vi "Get All Sub-Entries.vi"(8 "Error In":errorcluster, 11 "reference in":refnum<class "OD Entry.lvclass">) -> (0 "Error Out":errorcluster, 1 "Indices":u8[](array[numeric]), 2 "Sub-Entries":refnum<class "OD Sub-Entry.lvclass">[](array[class]), 3 "reference out":refnum<class "OD Entry.lvclass">)   [LabVIEW 2020, in "Electronic Datasheet.lvlib" / "OD Entry.lvclass"]
uses:
  OD Entry.lvclass
  OD Sub-Entry/OD Sub-Entry.lvclass
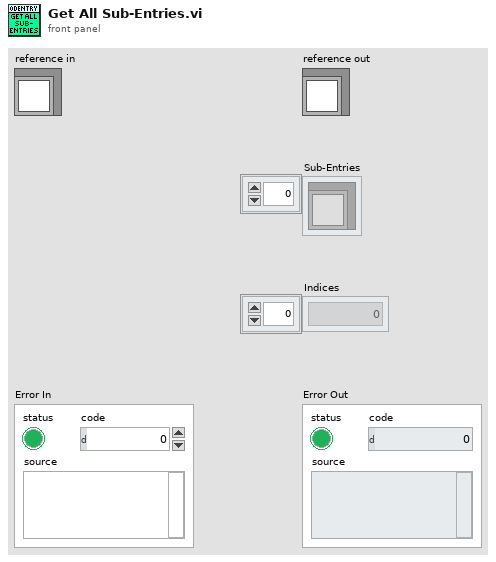
[diagram p1: front panel]
types:
  T1 = typedef "Electronic Datasheet.lvlib/OD Entry.lvclass/ObjectAttributes.ctl" = cluster{"Index":u16, "ObjectType":refnum<class "Object Type Base.lvclass">, "Denotation":string, "Count":u8, "ObjExtend":u8, "Label":string, "Description":string, "PDO Mapping Type":T2, "Sub-Entries":map{u8, refnum<class "OD Sub-Entry.lvclass">}}
  T2 = typedef "Electronic Datasheet.lvlib/PDO Mapping Type.ctl" = enum16{"no", "optional", "RPDO", "TPDO", "UNKNOWN"}
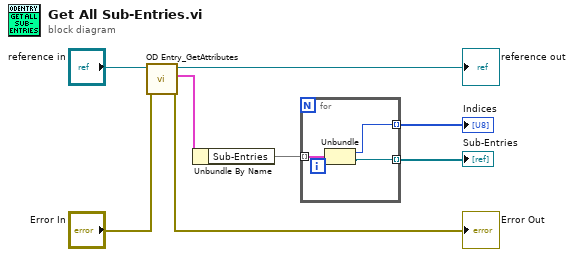
[diagram p0: block diagram]
diagram:
  n1 = call "OD Entry_GetAttributes.vi"("Error In"="Error In", "reference in"="reference in") -> ("Error Out"=→"Error Out":errorcluster, "Data"=w4:T1, "reference out"=→"reference out":refnum<class "OD Entry.lvclass">)  [unwired: 6 in, 1 out]
  n2 = Unbundle By Name(w4) -> ("Sub-Entries"=w3:map{u8, refnum<class "OD Sub-Entry.lvclass">})
  n3 = for {
    tunnel: w3 -> [w11] mode=indexing
    tunnel: [w10] -> w2 mode=indexing
    tunnel: [w9] -> w1 mode=indexing
    n4 = Unbundle(w11) -> ("Sub-Index"=w10:u8, "OD Sub-Entry"=w9:refnum<class "OD Sub-Entry.lvclass">)
  }
  "Sub-Entries" <- w1
  "Indices" <- w2
